vi "UART Write.vi"(8 "Error In":errorcluster, 10 "Data":string, 11 "ChipKit Resource 2":T1={"COM Port"="", "Board Type"=enum."ChipKit uC32", "Connection Type"=enum."USB / Serial", "Baud Rate (115200)"=15, "Bytes Per Packet (15)"=15}) -> (0 "Error Out":errorcluster, 3 "ChipKit Resource":T1={"COM Port"="", "Board Type"=enum."ChipKit uC32", "Connection Type"=enum."USB / Serial", "Baud Rate (115200)"=15, "Bytes Per Packet (15)"=15})   [LabVIEW 2011, in "LabVIEW Interface for ChipKit.lvlib"]
uses:
  LabVIEW Interface for ChipKit.lvlib
  Private/Type Defs/Chipkit Resource.ctl
  Private/Type Defs/Board Type.ctl
  Private/Type Defs/Connection Type.ctl
  Private/Type Defs/Command.ctl
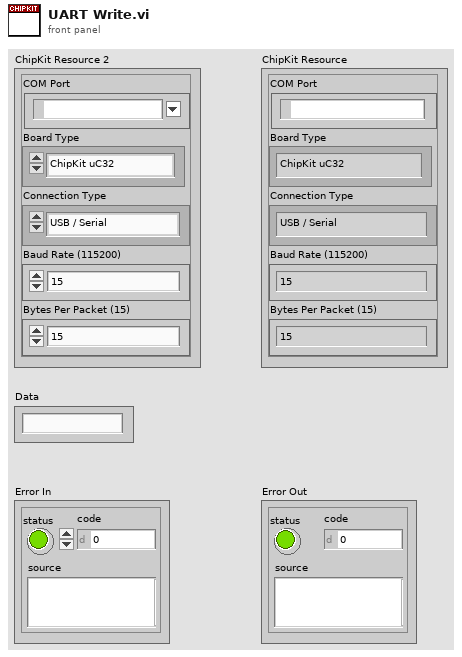
[diagram p1: front panel]
types:
  T1 = typedef "LabVIEW Interface for ChipKit.lvlib/Chipkit Resource.ctl" = cluster{"COM Port":refnum<visa-resource-name>, "Board Type":T2, "Connection Type":T3, "Baud Rate (115200)":u32, "Bytes Per Packet (15)":u32}
  T2 = typedef "LabVIEW Interface for ChipKit.lvlib/Board Type.ctl" = enum16{"ChipKit uC32", "ChipKit Uno32", "ChipKit Max32"}
  T3 = typedef "LabVIEW Interface for ChipKit.lvlib/Connection Type.ctl" = enum8{"USB / Serial", "XBEE", "BlueSmirf (Bluetooth)"}
  T4 = typedef "LabVIEW Interface for ChipKit.lvlib/Command.ctl" = enum8{"setArduinoMode", "flushSerial", "setPinMode", "digitalWritePin", "digitalWritePort", "tone", "digitalReadPin", "digitalReadPort", "analogReadPin", "analogReadPort", "pwmWritePin", "pwmWritePort", "sevenSegment_Configure", "sevenSegment_Write", "I2C Init", "I2C Write", "I2C Read", "SPI Init", "SPI Set Bit Order", "SPI Set Clock Divider", "SPI Set Data Mode", "SPI Send / Receive", "SPI Close", "Servo Set Num Servos", "Servo Config Servo", "Servo Write Angle", "Servo Read Angle", "Servo Write Pulse Width", "Servo Read Pulse Width", "Servo Detach", "LCD Init", "LCD Set Size", "LCD Set Cursor Mode", "LCD Clear", "LCD Set Cursor Position", "LCD Print", "LCD Display Power", "LCD Scroll Display", "LCD Autoscroll", "LCD Print Direction", "LCD Create Custom Char", "LCD Print Custom Char", "contAcqOn", "contAcqOff", "getFirmwareVersion", "FiniteSampleStart", "Reserved", "Reserved2", "Config Stepper", "Stepper Write", "Steper Detach", "Stepper Steps To Go", "UART Open", "UART Write", "UART Bytes Available", "UART Read"}
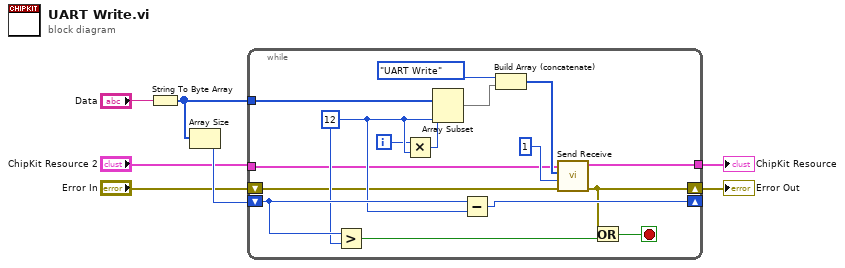
[diagram p0: block diagram]
diagram:
  n1 = String To Byte Array(string="Data") -> (unsigned byte array=w6:u8[])
  n2 = Array Size(array=w6) -> (size(s)=w5:i32)
  n3 = while {
    tunnel: w6 -> [w18]
    shift-right: [w13] -> _
    shift-left: w5 -> [w15]
    shift-right: [w10] -> w1
    shift-left: "Error In" -> [w11]
    tunnel: "ChipKit Resource 2" -> [w9]
    tunnel: [w8] -> w2
    i -> [w12]
    stop <- w19 stop-if-true
    w14 = 12 ("y")
    n4 = Greater?(x=w15, y=w14) -> (0:w20:bool)
    n5 = Multiply(x=w12, y=w14) -> (x*y=w17:i32)
    n6 = Array Subset(array=w18, index=w17, length=w14) -> (w16:u8[])
    n7 = Subtract(x=w15, y=w14) -> (x-y=w13:i32)
    n8 = Build Array (concatenate)(Command."UART Write" ("Command"), w16) -> (w22:u8[])
    n9 = call "Send Receive.vi"("Error In"=w11, "Bytes To Read (0)"=u32 1, "Data"=w22, "ChipKit Resource"=w9) -> ("Error Out"=w10:errorcluster, "ChipKit Resource"=w8:T1)  [unwired: 5 in, 1 out]
    n10 = Or(x=w10, y=w20) -> (x .or. y?=w19:bool)
  }
  "Error Out" <- w1
  "ChipKit Resource" <- w2
